vi "Actor Core.vi"(8 "error in":errorcluster, 11 "State in":refnum<class "Driver.lvclass">) -> (0 "error out":errorcluster, 3 "Actor out":refnum<class "Actor.lvclass">)   [LabVIEW 2014, in "Driver.lvlib" / "Driver.lvclass"]
doc: "(<B>Filename</B>: Actor Framework.lvlib:Actor.lvclass:Actor Core.vi)\n\nThis override invokes Entry.vi on the initial state, prior to calling the parent Actor Core. Adding this behavior to Actor Core (instead of an override of Pre Launch Init.vi) allows the initial state to launch a nested actor as part of its entry behavior.\n\nReceives messages to the actor, reacts to them, and initiates any error handling that may shut the actor down.\n\nDescendant classes may override this VI to append parallel tasks for the actor to complete while it handles messages. Overrides use the Call Parent Method node."
uses:
  Driver.lvclass
  <vilib>/ActorFramework/Actor/Actor.lvclass
  Driver State.ctl
  Joystick/Joystick Class/Button State.ctl
  Joystick/Joystick Class/Axis State.ctl
  Driver Messages/Get Driver Joystick State Msg/Get Driver Joystick State Msg.lvclass
  Driver.lvclass/Driver.ctl
  Joystick/Joystick Class/Joystick.lvclass
  Robot Actor Framework/System Actor/System Actor Class/System Actor.lvclass
panel:
  in  "Driver State":T1 {"Slide Right Joystick" min=-1.0 max=1.0 scale=-1.0..1.0; "Rotate Right Joystick" min=-1.0 max=1.0 scale=-1.0..1.0; "Forward Joystick" min=-1.0 max=1.0 scale=-1.0..1.0}
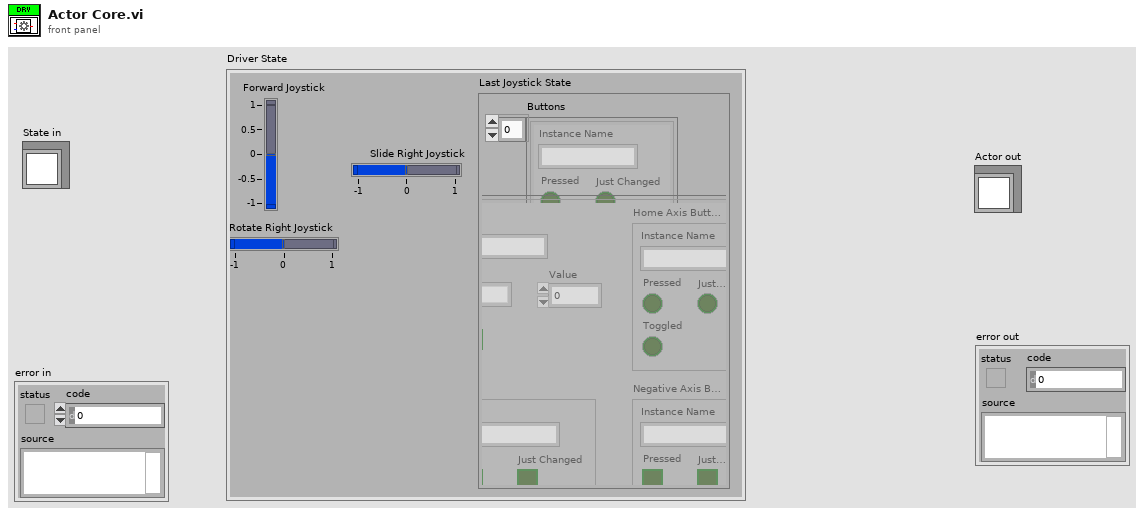
[diagram p1: front panel]
types:
  T1 = typedef "Driver.lvlib/Driver.lvclass/Driver State.ctl" = cluster{"Forward Joystick":dbl, "Rotate Right Joystick":dbl, "Slide Right Joystick":dbl, "Last Joystick State":cluster{"Buttons":T2[], "Axis":T3[]}}
  T2 = typedef "Joystick.lvlib/Joystick.lvclass/Button State.ctl" = cluster{"Pressed":bool, "Instance Name":string, "Toggled":bool, "Just Changed":bool}
  T3 = typedef "Joystick.lvlib/Joystick.lvclass/Axis State.ctl" = cluster{"Instance Name":string, "Deadband":dbl, "Value":dbl, "At Home":bool, "Postive Axis Button State":T2, "Negative Axis Button State":T2, "Home Axis Button State":T2}
  T4 = enum16{"Critical", "Error", "Warning", "Informational", "Debug"}
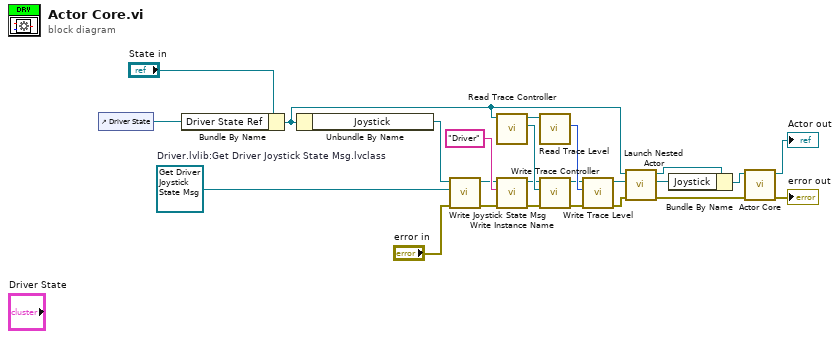
[diagram p0: block diagram]
diagram:
  w3 = refnum<class "Get Driver Joystick State Msg.lvclass"> refnum  # Driver.lvlib:Get Driver Joystick State Msg.lvclass
  n1 = control-ref of="Driver State"() -> (w17:refnum<vi>)
  n2 = Bundle By Name(cluster="State in", "Driver State Ref"=w17) -> (w14:refnum<class "Driver.lvclass">)
  n3 = Unbundle By Name(w14) -> ("Joystick"=w5:refnum<class "Joystick.lvclass">)
  n4 = call-dynamic "Write Joystick State Msg.vi"("error in (no error)"="error in", "Joystick.lvlib:Get Joystick State Msg.lvclass"=w3, "Joystick in"=w5) -> ("error out"=w1:errorcluster, "Joystick out"=w4:refnum<class "Joystick.lvclass">)  [unwired: 7 in]
  n5 = call-dynamic "Read Trace Controller.vi"("System Actor in"=w14) -> ("Trace Controller"=w11:refnum<class "Message Enqueuer.lvclass">, "System Actor out"=w13:refnum<class "Driver.lvclass">)  [unwired: 8 in, 1 out]
  n6 = call-dynamic "Write Instance Name.vi"("error in (no error)"=w1, "Instance Name"="Driver", "System Actor in"=w4) -> ("error out"=w8:errorcluster, "System Actor out"=w9:refnum<class "Joystick.lvclass">)  [unwired: 7 in]
  n7 = call-dynamic "Read Trace Level.vi"("System Actor in"=w13) -> ("Trace Level"=w15:T4)  [unwired: 8 in, 2 out]
  n8 = call-dynamic "Write Trace Controller.vi"("error in (no error)"=w8, "Trace Controller"=w11, "System Actor in"=w9) -> ("error out"=w7:errorcluster, "System Actor out"=w12:refnum<class "Joystick.lvclass">)  [unwired: 7 in]
  n9 = call-dynamic "Write Trace Level.vi"("error in (no error)"=w7, "Trace Level"=w15, "System Actor in"=w12) -> ("error out"=w6:errorcluster, "System Actor out"=w16:refnum<class "Joystick.lvclass">)  [unwired: 7 in]
  n10 = call <vilib>:"Launch Nested Actor.vi"("error in (no error)"=w6, "Nested Actor"=w16, "Caller Actor in"=w14) -> ("error out"=w19:errorcluster, "Nested Actor's Enqueuer"=w20:refnum<class "Message Enqueuer.lvclass">, "Caller Actor out"=w22:refnum<class "Driver.lvclass">)  [unwired: 6 in]
  n11 = Bundle By Name(cluster=w22, "Joystick"=w20) -> (w21:refnum<class "Driver.lvclass">)
  n12 = call-parent "Actor Core.vi"("error in"=w19, "State in"=w21) -> ("error out"=→"error out":errorcluster, "Actor out"=→"Actor out":refnum<class "Actor.lvclass">)  [unwired: 8 in]
